vi "neuron.vi"(1 "Weights":dbl[](array[numeric]), 2 "Inputs":dbl[](array[numeric]), 3 "Function":u16(ring) items=["Siqmoid", "Linear", "Sign"]) -> (0 "Output":dbl)   [LabVIEW 2009]
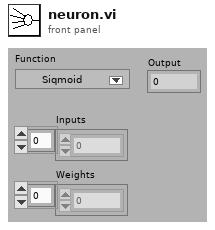
[diagram p1: front panel]
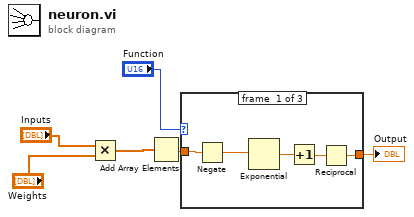
[diagram p0: block diagram]
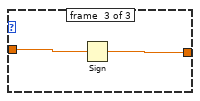
[diagram p3: hidden frame]
diagram:
  n1 = Multiply(x="Inputs", y="Weights") -> (x*y=w6:dbl[])
  n2 = Add Array Elements(numeric array=w6) -> (sum=w5:dbl)
  n3 = case shown="0, Default" "Function" {
    tunnel: w5 -> [w8 w12 w14]
    tunnel: [w7 w12 w13] -> w4
    frame #0 {
      n4 = Negate(x=w8) -> (-x=w11:dbl)
      n5 = Exponential(1:w11) -> (0:w10:dbl)
      n6 = Increment(x=w10) -> (x+1=w9:dbl)
      n7 = Reciprocal(x=w9) -> (1/x=w7:dbl)
    }
    frame #1 {
    }
    frame #2 {
      n8 = Sign(1:w14) -> (0:w13:dbl)
    }
  }
  "Output" <- w4
